vi "(auto) Go back Action.vi"(5 "I2C Ref in":T1, 11 "BackState":enum16{"0", "1", "2", "3", "4", "5", "6", ""}(ring)) -> (2 "I2C Ref Out":T1)   [LabVIEW 2017]
uses:
  <vilib>/myRIO/Instrument Drivers/Onboard IO/I2C/typedefs/I2C Reference.ctl
  <vilib>/myRIO/Common/Instrument Driver Framework/Utilities/typedefs/myRIO Generic Hardware Reference.ctl
  <vilib>/myRIO/Common/Instrument Driver Framework/Utilities/typedefs/Hardware Version Enum.ctl
  <vilib>/myRIO/Common/Instrument Driver Framework/Utilities/typedefs/myRIO v1.0 Reference.ctl
  <vilib>/myRIO/Common/Instrument Driver Framework/Utilities/typedefs/Generic FPGA Reference.ctl
  <vilib>/myRIO/Common/Instrument Driver Framework/myRIO v1.0/I2C/typedefs/I2C Channels Enum.ctl
  <vilib>/myRIO/Instrument Drivers/Onboard IO/I2C/typedefs/I2C Configuration.ctl
  <vilib>/myRIO/Instrument Drivers/Onboard IO/I2C/typedefs/I2C Transfer Rate.ctl
  <vilib>/myRIO/Instrument Drivers/Onboard IO/I2C/I2C.lvlib
panel:
  in  "M_UB":i32
  in  "G_UB":i32
  in  "M_UB 2":i32
  in  "G_UB 2":i32
  in  "Stop Button":bool
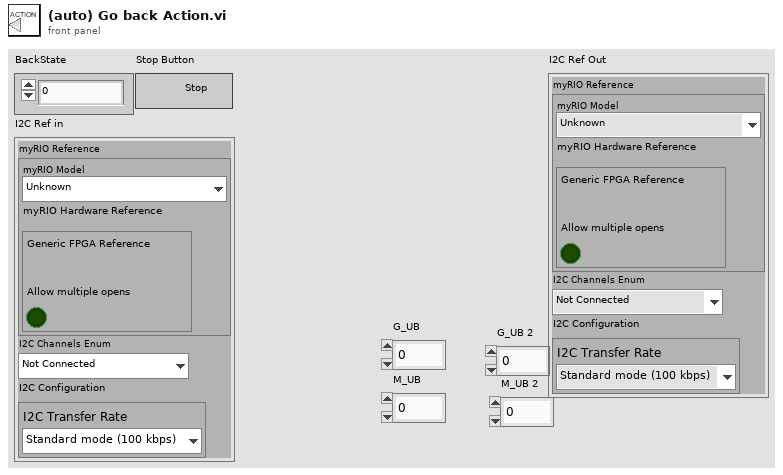
[diagram p1: front panel]
types:
  T1 = typedef "I2C.lvlib/I2C Reference.ctl" = cluster{"myRIO Reference":T2, "I2C Channels Enum":T6, "I2C Configuration":T7}
  T2 = typedef "myRIO Generic Hardware Reference.ctl" = cluster{"myRIO Model":T3, "myRIO Hardware Reference":T4}
  T3 = typedef "Hardware Version Enum.ctl" = enum16{"Unknown", "myRIO-1900", "myRIO-1950", "roboRIO", "NI ELVIS RIO CM"}
  T4 = typedef "myRIO v1.0 Reference.ctl" = cluster{"Generic FPGA Reference":T5, "Allow multiple opens":bool}
  T5 = typedef "Generic FPGA Reference.ctl" = refnum<k20>
  T6 = typedef "I2C Channels Enum.ctl" = enum16{"Not Connected", "A/I2C", "B/I2C", "I2C/I2C"}
  T7 = typedef "I2C.lvlib/I2C Configuration.ctl" = cluster{"I2C Transfer Rate":T8}
  T8 = typedef "I2C.lvlib/I2C Transfer Rate.ctl" = enum16{"Standard mode (100 kbps)", "Fast mode (400 kbps)"}
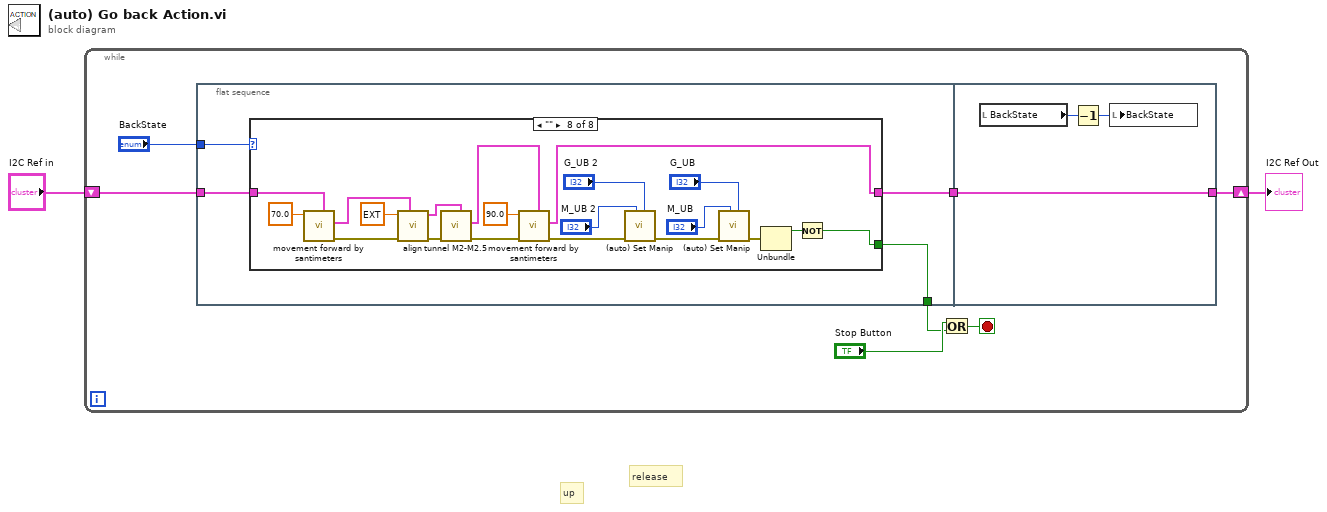
[diagram p0: block diagram]
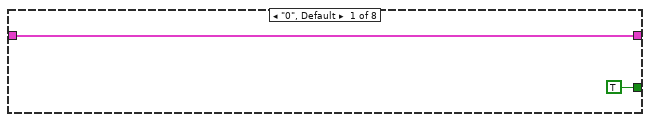
[diagram p2: hidden frame]
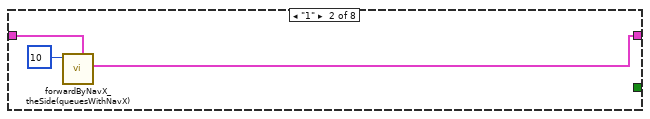
[diagram p3: hidden frame]
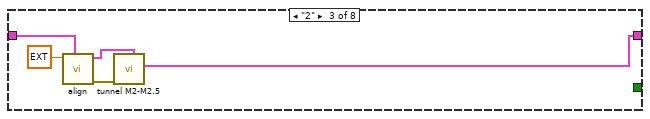
[diagram p4: hidden frame]
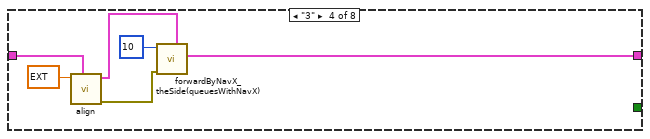
[diagram p5: hidden frame]
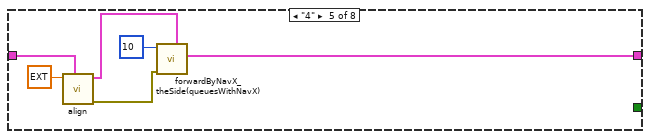
[diagram p6: hidden frame]
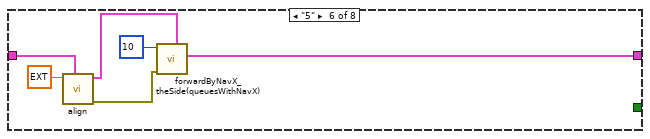
[diagram p7: hidden frame]
diagram:
  # "release"
  # "up"
  n1 = while {
    shift-right: [w7] -> w1
    shift-left: "I2C Ref in" -> [w8]
    stop <- w6 stop-if-true
    n2 = flat-sequence {
      tunnel: "BackState" -> [w13]
      tunnel: w8 -> [w12]
      tunnel: [w10] -> w4
      tunnel: [w11] -> w3
      tunnel: [w65] -> w7
      tunnel: w3 -> [w65]
      frame #0 {
        n3 = case shown="\"\"" w13 {
          tunnel: [w15 w16 w19 w24 w30 w36 w42 w43] -> w11
          tunnel: w12 -> [w15 w17 w21 w28 w34 w38 w42 w55]
          tunnel: [TRUE _ _ _ _ _ _ w57] -> w10
          frame "0", Default {
          }
          frame "1" {
            n4 = call "forwardByNavX_theSide(queuesWithNavX).vi"("I2C Ref Out"=w17, "distance the side"=u32 10) -> ("I2C Ref Out 2"=w16:T1)  [unwired: 8 in, 1 out]
          }
          frame "2" {
            n5 = call "align.vi"("I2C Ref Out"=w21, "Angle"=ext 90.0) -> ("error out"=w22:errorcluster, "I2C Ref Out out"=w20:T1)  [unwired: 7 in, 1 out]
            n6 = call "tunnel M2-M2.5.vi"("I2C Ref in"=w20, "error in (no error)"=w22) -> ("I2C Ref Out"=w19:T1)  [unwired: 8 in, 1 out]
          }
          frame "3" {
            n7 = call "align.vi"("I2C Ref Out"=w28, "Angle"=ext 180.0) -> ("error out"=w26:errorcluster, "I2C Ref Out out"=w25:T1)  [unwired: 7 in, 1 out]
            n8 = call "forwardByNavX_theSide(queuesWithNavX).vi"("I2C Ref Out"=w25, "error in (no error)"=w26, "distance the side"=u32 10) -> ("I2C Ref Out 2"=w24:T1)  [unwired: 7 in, 1 out]
          }
          frame "4" {
            n9 = call "align.vi"("I2C Ref Out"=w34, "Angle"=ext 90.0) -> ("error out"=w32:errorcluster, "I2C Ref Out out"=w31:T1)  [unwired: 7 in, 1 out]
            n10 = call "forwardByNavX_theSide(queuesWithNavX).vi"("I2C Ref Out"=w31, "error in (no error)"=w32, "distance the side"=u32 10) -> ("I2C Ref Out 2"=w30:T1)  [unwired: 7 in, 1 out]
          }
          frame "5" {
            n11 = call "align.vi"("I2C Ref Out"=w38, "Angle"=ext 90.0) -> ("error out"=w39:errorcluster, "I2C Ref Out out"=w37:T1)  [unwired: 7 in, 1 out]
            n12 = call "forwardByNavX_theSide(queuesWithNavX).vi"("I2C Ref Out"=w37, "error in (no error)"=w39, "distance the side"=u32 10) -> ("I2C Ref Out 2"=w36:T1)  [unwired: 7 in, 1 out]
          }
          frame "6" {
          }
          frame "" {
            n13 = call "movement forward by santimeters.vi"("I2C Ref in"=w55, "distance (cm)"=70.0) -> ("error out"=w61:errorcluster, "I2C Ref out"=w54:T1)  [unwired: 8 in]
            n14 = call "align.vi"("I2C Ref Out"=w54, "error in (no error)"=w61, "Angle"=ext 90.0) -> ("error out"=w59:errorcluster, "I2C Ref Out out"=w56:T1)  [unwired: 6 in, 1 out]
            n15 = call "tunnel M2-M2.5.vi"("I2C Ref in"=w56, "error in (no error)"=w59) -> ("error out"=w46:errorcluster, "I2C Ref Out"=w44:T1)  [unwired: 8 in]
            n16 = call "movement forward by santimeters.vi"("I2C Ref in"=w44, "error in (no error)"=w46, "distance (cm)"=90.0) -> ("error out"=w52:errorcluster, "I2C Ref out"=w43:T1)  [unwired: 7 in]
            n17 = call "(auto) Set Manip.vi"("G_upper bound"="G_UB 2", "M_lower bound"="M_UB 2", "error in (no error)"=w52) -> ("error out"=w49:errorcluster)  [unwired: 8 in]
            n18 = call "(auto) Set Manip.vi"("G_upper bound"="G_UB", "M_lower bound"="M_UB", "error in (no error)"=w49) -> ("error out"=w45:errorcluster)  [unwired: 8 in]
            n19 = Unbundle(w45) -> ("status"=w58:bool)  [unwired: 2 out]
            n20 = Not(x=w58) -> (.not. x?=w57:bool)
          }
        }
      }
      frame #1 {
        n21 = local read "BackState"() -> (w64:enum16{"0", "1", "2", "3", "4", "5", "6", ""})
        n22 = Decrement(x=w64) -> (x-1=w63:enum16{"0", "1", "2", "3", "4", "5", "6", ""})
        n23 = local write "BackState"(w63) -> ()
      }
    }
    n24 = Or(x="Stop Button", y=w4) -> (x .or. y?=w6:bool)
  }
  "I2C Ref Out" <- w1
